vi "Basic Obstacle avoiding ui.vi"() -> ()   [LabVIEW 2022 SP3]
panel:
  out "error out":errorcluster
  in  "byte count":u32=4
  out "read buffer":string
  in  "VISA resource name":refnum<visa-resource-name>
  out "Safe Zone":bool
  out "Caution Zone":bool
  out "Critical zone":bool
  in  "stop":bool
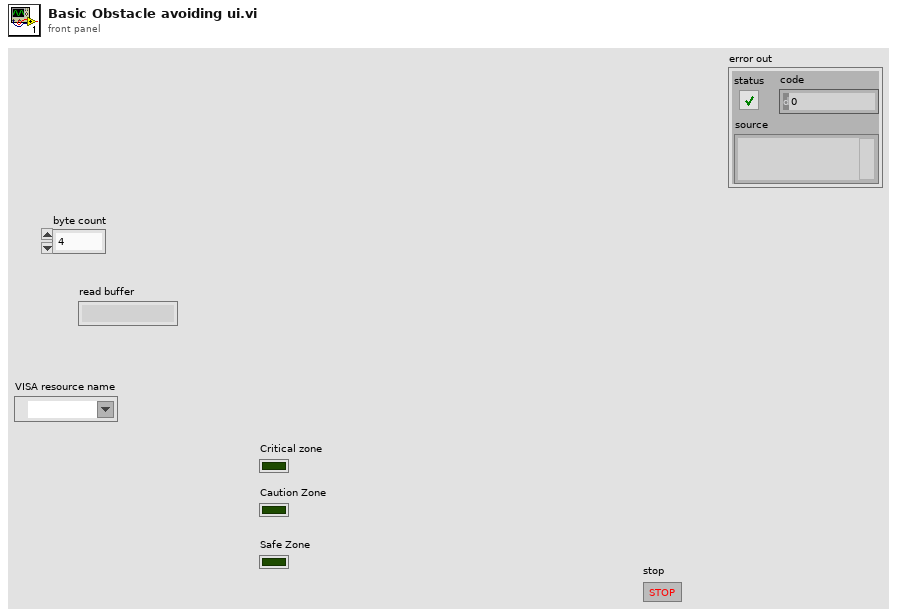
[diagram p1: front panel]
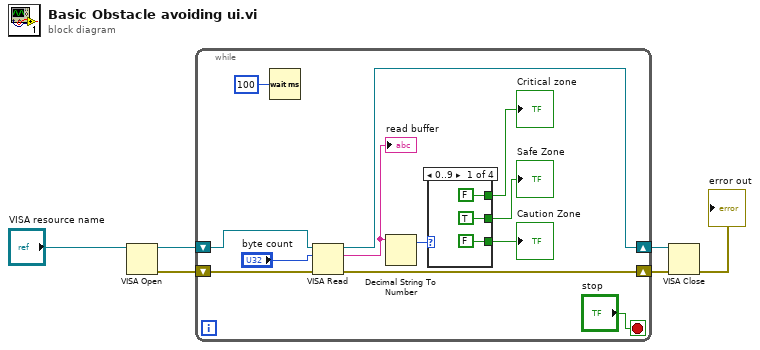
[diagram p0: block diagram]
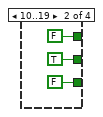
[diagram p2: hidden frame]
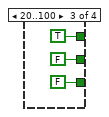
[diagram p3: hidden frame]
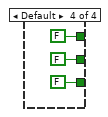
[diagram p4: hidden frame]
diagram:
  n1 = VISA Open(VISA resource name="VISA resource name") -> (VISA resource name=w6:refnum<visa-resource-name>, error out=w4:errorcluster)  [unwired: 4 in]
  n2 = while {
    shift-right: [w12] -> w5
    shift-left: w6 -> [w13]
    shift-right: [w10] -> w3
    shift-left: w4 -> [w11]
    stop <- "stop" stop-if-true
    n3 = Wait (ms)(milliseconds to wait=u32 100) -> ()  [unwired: 1 out]
    n4 = VISA Read(VISA resource name=w13, byte count="byte count", error in (no error)=w11) -> (VISA resource name out=w12:refnum<visa-resource-name>, read buffer=w9:string, error out=w10:errorcluster)  [unwired: 1 out]
    "read buffer" <- w9
    n5 = Decimal String To Number(string=w9) -> (offset past number=w8:i32)  [unwired: 2 in, 1 out]
    n6 = case shown="0..9" w8 {
      tunnel: [FALSE ("Critical zone") FALSE ("Critical zone") TRUE ("Critical zone") FALSE ("Critical zone")] -> w16
      tunnel: [FALSE ("Caution Zone") FALSE ("Caution Zone") FALSE ("Caution Zone") FALSE ("Caution Zone")] -> w15
      tunnel: [TRUE ("Safe Zone") TRUE ("Safe Zone") FALSE ("Safe Zone") FALSE ("Safe Zone")] -> w14
      frame 0..9 {
      }
      frame 10..19 {
      }
      frame 20..100 {
      }
      frame Default {
      }
    }
    "Critical zone" <- w16
    "Caution Zone" <- w15
    "Safe Zone" <- w14
  }
  n7 = VISA Close(VISA resource name=w5, error in (no error)=w3) -> (error out=→"error out":errorcluster)
